vi "EmailSender.vi"() -> ()   [LabVIEW 2024]
uses:
  <vilib>/smtpClient/SmtpClientHandle.ctl
  <vilib>/smtpClient/Set Message Text.vi
  <vilib>/smtpClient/LabVIEWSMTPClient.lvlib
panel:
  out "invalid recipients":string[](array[string])
  out "handle out":T1
  out "error out":errorcluster
  in  "to":string[](array[string])
  in  "attachments":path[](array[path])
  in  "plain text message":string
  in  "subject":string
  in  "password":string
  in  "from":string
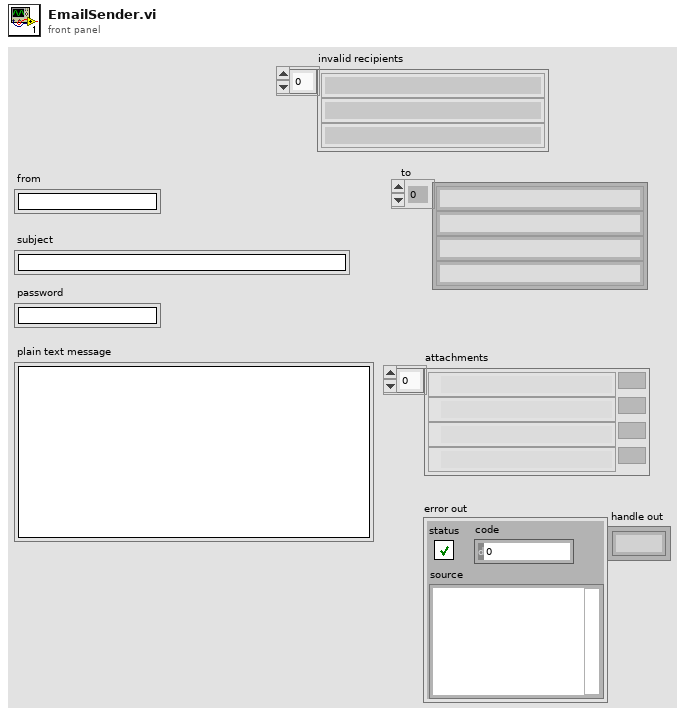
[diagram p1: front panel]
types:
  T1 = typedef "LabVIEWSMTPClient.lvlib/SmtpClientHandle.ctl" = refnum<k1>
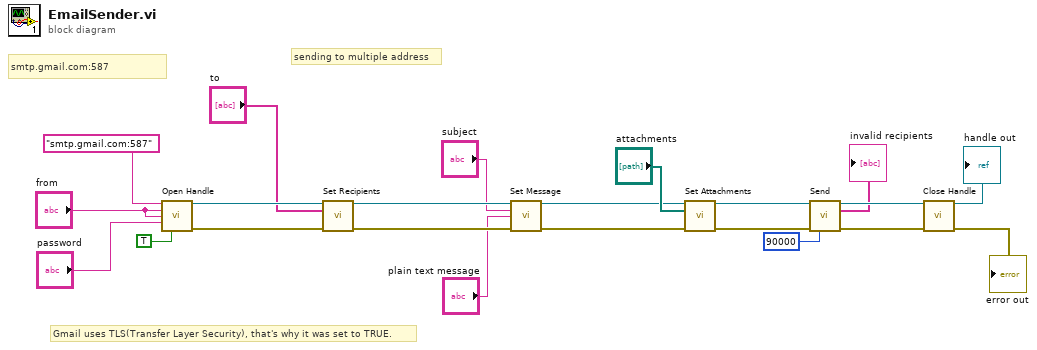
[diagram p0: block diagram]
diagram:
  # "Gmail uses TLS(Transfer Layer Security), that's why it was set to TRUE."
  # "sending to multiple address"
  # "smtp.gmail.com:587"
  n1 = call <vilib>:"Open Handle.vi"("server address"="smtp.gmail.com:587", "from"="from", "username"="from", "password"="password", "use TLS (false)"=TRUE) -> ("handle out"=w22:T1, "error out"=w19:errorcluster)  [unwired: 9 in]
  n2 = call <vilib>:"Set Recipients.vi"("handle in"=w22, "to"="to", "error in (no error)"=w19) -> ("handle out"=w21:T1, "error out"=w18:errorcluster)  [unwired: 11 in]
  n3 = call-poly <vilib>:"Set Message.vi"("handle in"=w21, "subject"="subject", "plain text message"="plain text message", "error in (no error)"=w18) -> ("handle out"=w10:T1, "error out"=w9:errorcluster)  [unwired: 10 in]
  n4 = call <vilib>:"Set Attachments.vi"("handle in"=w10, "attachments"="attachments", "error in (no error)"=w9) -> ("handle out"=w7:T1, "error out"=w8:errorcluster)  [unwired: 11 in]
  n5 = call <vilib>:"Send.vi"("handle in"=w7, "error in (no error)"=w8, "timeout in ms (10000)"=90000) -> ("handle out"=w20:T1, "invalid recipients"=→"invalid recipients":string[], "error out"=w17:errorcluster)  [unwired: 10 in]
  n6 = call <vilib>:"Close Handle.vi"("handle in"=w20, "error in (no error)"=w17) -> ("handle out"=→"handle out":T1, "error out"=→"error out":errorcluster)  [unwired: 12 in]
